vi "总磷总氮报警信息.vi"(8 "error in (no error)":errorcluster, 11 "data in":T1) -> (0 "error out":errorcluster)   [LabVIEW 2016, in "斯坦道总磷总氮.lvlib"]
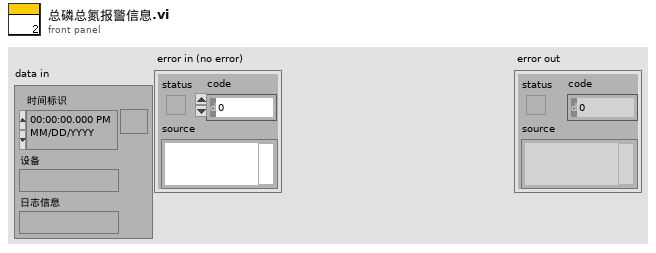
[diagram p1: front panel]
types:
  T1 = cluster{"时间标识":timestamp, "设备":string, "日志信息":string}
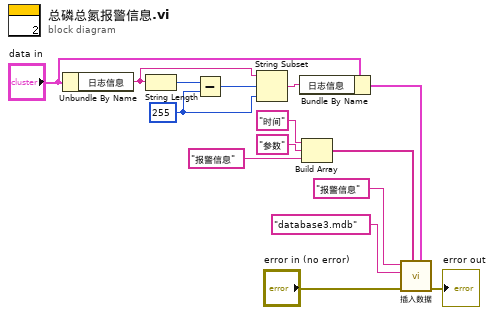
[diagram p0: block diagram]
diagram:
  w4 = 255 ("y")
  n1 = Unbundle By Name("data in") -> ("日志信息"=w7:string)
  n2 = String Length(string=w7) -> (length=w6:i32)
  n3 = Subtract(x=w6, y=w4) -> (x-y=w5:i32)
  n4 = String Subset(string=w7, offset (0)=w5, length (rest)=w4) -> (substring=w2:string)
  n5 = Bundle By Name(cluster="data in", "日志信息"=w2) -> (w1:T1)
  n6 = Build Array("时间", "参数" ("元素"), "报警信息") -> (w12:string[])
  n7 = call "插入数据.vi"("data"=w1, "columns"=w12, "error in (no error)"="error in (no error)", "database"="database3.mdb", "table"="报警信息") -> ("error out"=→"error out":errorcluster)  [unwired: 6 in]
